vi "字符串转时间.vi"(11 "时间字符串":string="2015/7/10 14:34:23") -> (3 "时间标识":timestamp)   [LabVIEW 2014]
uses:
  <vilib>/Utility/miscctls.llb/LVDateTimeRec.ctl
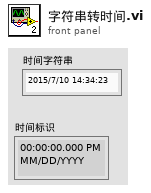
[diagram p1: front panel]
types:
  T1 = typedef "LVDateTimeRec.ctl" = cluster{"fractional second":dbl, "second":i32, "minute":i32, "hour":i32, "day of month":i32, "month":i32, "year":i32, "day of week":i32, "day of year":i32, "DST":i32}
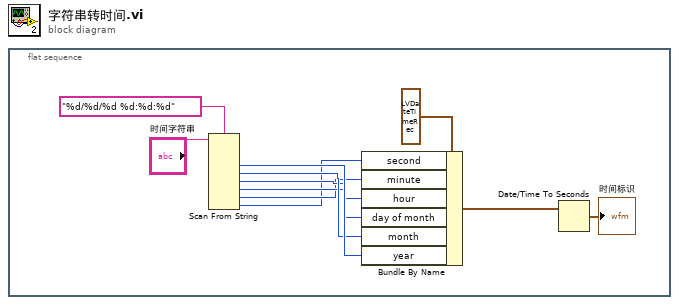
[diagram p0: block diagram]
diagram:
  n1 = flat-sequence {
    frame #0 {
      n2 = Scan From String(format string="%d/%d/%d %d:%d:%d" ("格式字符串"), input string="时间字符串") -> (output 1=w7:i32, output 2=w6:i32, output 3=w5:i32, output 4=w4:i32, output 5=w3:i32, output 6=w2:i32)  [unwired: 8 in, 3 out]
      n3 = Bundle By Name(cluster=T1 {"fractional second"=0.0, "second"=0, "minute"=0, "hour"=0, "day of month"=0, "month"=0, "year"=0, "day of week"=0, "day of year"=0, "DST"=0} ("日期时间记录"), "second"=w2, "minute"=w3, "hour"=w4, "day of month"=w5, "month"=w6, "year"=w7) -> (w1:T1)
      n4 = Date/Time To Seconds(2:w1) -> (0:→"时间标识":timestamp)  [unwired: 1 in]
    }
  }
